vi "Renishaw-XL80_SetLambda.vi"(8 "error in (no error)":errorcluster, 10 "Lambda":dbl, 11 "Renishaw-XL80 in":refnum<class "Renishaw-XL80.lvclass">) -> (0 "error out":errorcluster, 3 "Renishaw-XL80 out":refnum<class "Renishaw-XL80.lvclass">)   [LabVIEW 2024, in "Renishaw-XL80.lvclass"]
doc: "Lambda property\nWriting this property will set the wavelength in µm.\n\nDefinition\nHRESULTput_Lambda( [in] double newVal);\nParameters\nnewVal\nSpecifies the wavelength to use (in µm).\n\nComments\nThis property will return with an HRESULT of E_FAIL if the client has not set AutoCompensationMode to AUTO_COMPENSATION_OFF. This warns the client that setting lambda whilst it is being automatically updated is somewhat pointless. Otherwise the property will return an HRESULT of S_OK.\n\n\nSee Also"
uses:
  Renishaw-XL80.lvclass
  Renishaw-XL80.lvclass/Renishaw-XL80.ctl
  D:/A.C.M/Example CSharp_64/bin/Debug/Interop.DX10SDKADAPTORLib.dll
  Example CSharp_64/bin/Debug/Interop.DX10SDKADAPTORLib.dll
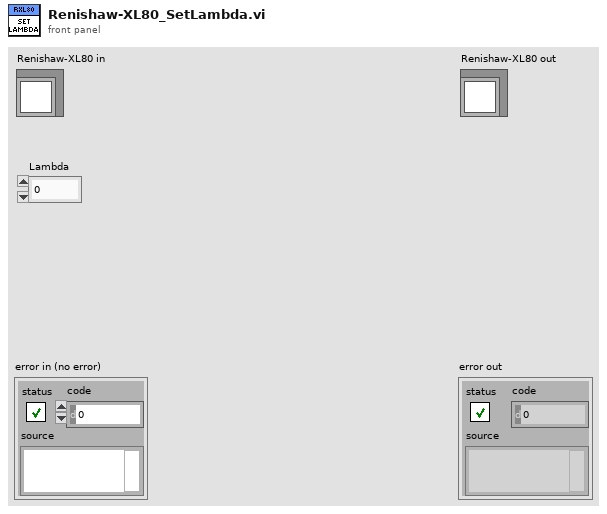
[diagram p1: front panel]
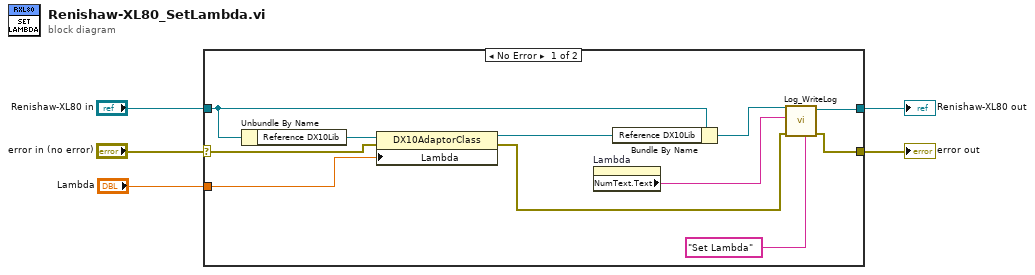
[diagram p0: block diagram]
diagram:
  n1 = case shown="No Error" "error in (no error)" {
    selector: "error in (no error)" -> [w14 w18]
    tunnel: [w9 w18] -> w4
    tunnel: [w11 w17] -> w2
    tunnel: "Renishaw-XL80 in" -> [w15 w17]
    tunnel: "Lambda" -> [w13 _]
    frame No Error {
      n2 = Unbundle By Name(w15) -> ("Reference DX10Lib"=w7:refnum<k24>)
      n3 = property class="DX10AdaptorClass"(reference=w7, error in=w14, "Lambda"=w13) -> (reference out=w16:refnum<k24>, error out=w6:errorcluster)
      n4 = property on="Lambda" class="DigNum (strict)"() -> ("NumText.Text"=w10:string)  [unwired: 2 in, 2 out]
      n5 = Bundle By Name(cluster=w15, "Reference DX10Lib"=w16) -> (w12:refnum<class "Renishaw-XL80.lvclass">)
      n6 = call-dynamic "Log_WriteLog.vi"("Additional text"="Set Lambda", "error in (no error)"=w6, "Command"=w10, "Log in"=w12) -> ("error out"=w9:errorcluster, "Log out"=w11:refnum<class "Renishaw-XL80.lvclass">)  [unwired: 6 in]
    }
    frame Error {
    }
  }
  "error out" <- w4
  "Renishaw-XL80 out" <- w2
